vi "test_Write Pattern.vi"(8 "error in (no error)":errorcluster, 10 "IO Lines Patttern Settings":T2[](array[typedef]) {"Duration (us)" min=0.005 max=42550000.0 step=0.005 format="%#.3f"}, 11 "IO Lines Enable":T1={"Enable"=[FALSE, FALSE, FALSE, FALSE, FALSE, FALSE, FALSE, FALSE, FALSE, FALSE, FALSE, FALSE, FALSE, FALSE, FALSE, FALSE, FALSE, FALSE, FALSE, FALSE, FALSE, FALSE, FALSE, FALSE, FALSE, FALSE, FALSE, FALSE, FALSE, FALSE, FALSE, FALSE]}) -> (0 "error out":errorcluster, 2 "Pattern Digital Data":digitaldata, 3 "Data out":u64[](array[numeric])=[5631702913073631, 5629503829180420, 5629508124147720, 5629503829180426, 5629508124147722, 5629503829180426, 5629508124147722, 5629503829180426, 5629508124147722, 5631707147403291])   [LabVIEW 2016]
uses:
  Host/Typedefs/IO Lines State.ctl
  Host/Typedefs/IO Lines Enable.ctl
  Host/Typedefs/LV2G Operation.ctl
  Host/Typedefs/IO Buffer Operation.ctl
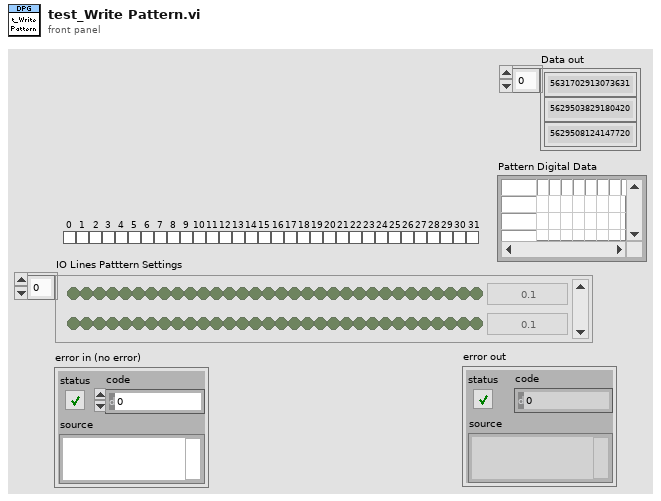
[diagram p1: front panel]
types:
  T1 = typedef "IO Lines Enable.ctl" = cluster{"Enable":bool[]}
  T2 = typedef "IO Lines State.ctl" = cluster{"State":bool[], "Duration (us)":dbl}
  T3 = typedef "IO Buffer Operation.ctl" = enum16{"Initialize", "Write IO Data_Rd", "Read IO Data_Rd", "Write IO Data_Wr", "Read IO Data_Wr", "Write  IO Data_Dir", "Read  IO Data_Dir", "Write Host to Target FIFO", "Read Host to Target FIFO", "Write Target to Host FIFO", "Read Target to Host FIFO", "Write Monitor Enable?", "Read Monitor Enable?", "Close"}
  T4 = typedef "LV2G Operation.ctl" = enum16{"Initialize", "Set", "Get", "Close"}
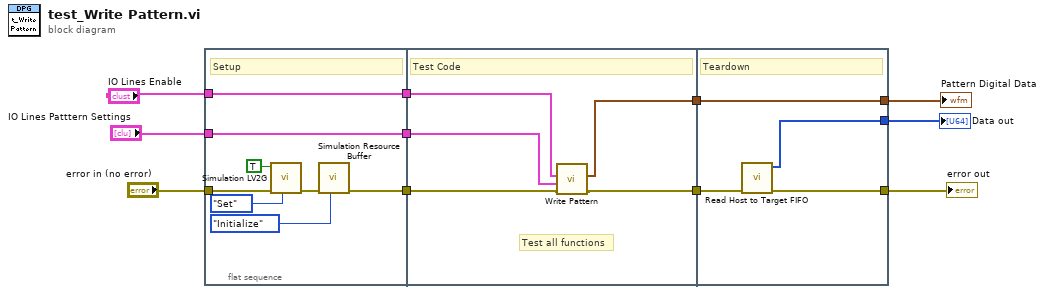
[diagram p0: block diagram]
diagram:
  n1 = flat-sequence {
    tunnel: "error in (no error)" -> [w19]
    tunnel: [w14] -> w11
    tunnel: [w13] -> w6
    tunnel: "IO Lines Patttern Settings" -> [w13]
    tunnel: "IO Lines Enable" -> [w12]
    tunnel: [w12] -> w1
    tunnel: w11 -> [w24]
    tunnel: [w23] -> w10
    tunnel: w6 -> [w22]
    tunnel: [w20] -> w4
    tunnel: w1 -> [w21]
    tunnel: [w27] -> w8
    tunnel: w10 -> [w28]
    tunnel: [w26] -> w7
    tunnel: w4 -> [w25]
    tunnel: [w25] -> w3
    frame #0 {
      # "Setup"
      n2 = call "Simulation LV2G.vi"("Operation (Get)"=LV2G_Operation."Set", "error in (no error)"=w19, "Simulation?"=TRUE) -> ("error out"=w16:errorcluster)  [unwired: 7 in, 1 out]
      n3 = call "Simulation Resource Buffer.vi"("IO Buffer Operation"=IO_Buffer_Operation."Initialize", "error in (no error)"=w16) -> ("error out"=w14:errorcluster)  [unwired: 7 in, 2 out]
    }
    frame #1 {
      # "Test all functions"
      # "Test Code"
      n4 = call "Write Pattern.vi"("error in (no error)"=w24, "IO Lines Pattteen"=w22, "IO Lines Enable"=w21) -> ("error out"=w23:errorcluster, "Pattern Digital Data"=w20:digitaldata)  [unwired: 6 in, 1 out]
    }
    frame #2 {
      # "Teardown"
      n5 = call "Read Host to Target FIFO.vi"("error in (no error)"=w28) -> ("error out"=w27:errorcluster, "Host to Target FIFO"=w26:u64[])  [unwired: 9 in]
    }
  }
  "error out" <- w8
  "Data out" <- w7
  "Pattern Digital Data" <- w3
